vi "POST (Multipart).vi"(6 "timeout":i32=10000, 7 "output file":path, 8 "error in":errorcluster, 9 "data":T1[](array[typedef]), 10 "url":string, 11 "session in":refnum<class "Session.lvclass">) -> (0 "error out":errorcluster, 1 "body":string, 2 "headers":string, 3 "session out":refnum<class "Session.lvclass">, 4 "status code":u32)   [LabVIEW 2024, in "lib_NI_Advanced HTTP Client.lvlib" / "Session.lvclass"]
uses:
  Session.lvclass
  Multipart Data--cluster.ctl
  Session.lvclass/Session.ctl
  lvwebclient_64.dll
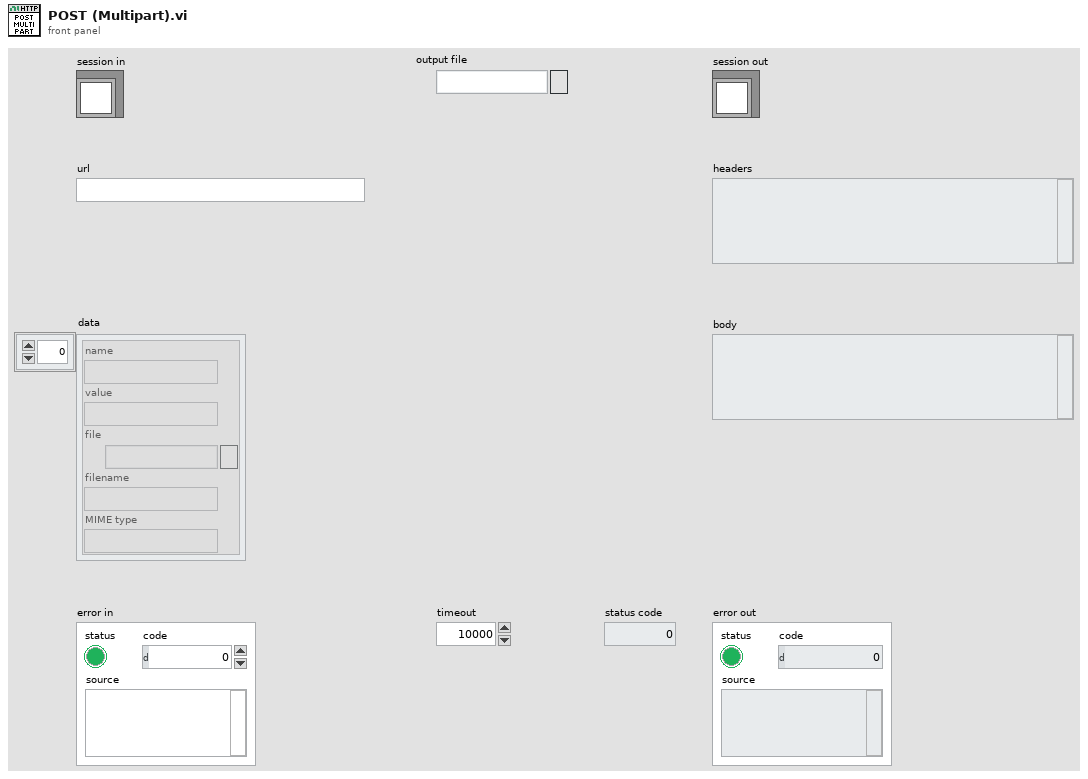
[diagram p1: front panel]
types:
  T1 = typedef "lib_NI_Advanced HTTP Client.lvlib/Session.lvclass/Multipart Data--cluster.ctl" = cluster{"name":string, "value":string, "file":path, "filename":string, "MIME type":string}
  T2 = cluster{"utf-8 text":string, "value":string, "file":path, "utf-8 text":string, "utf-8 text":string}
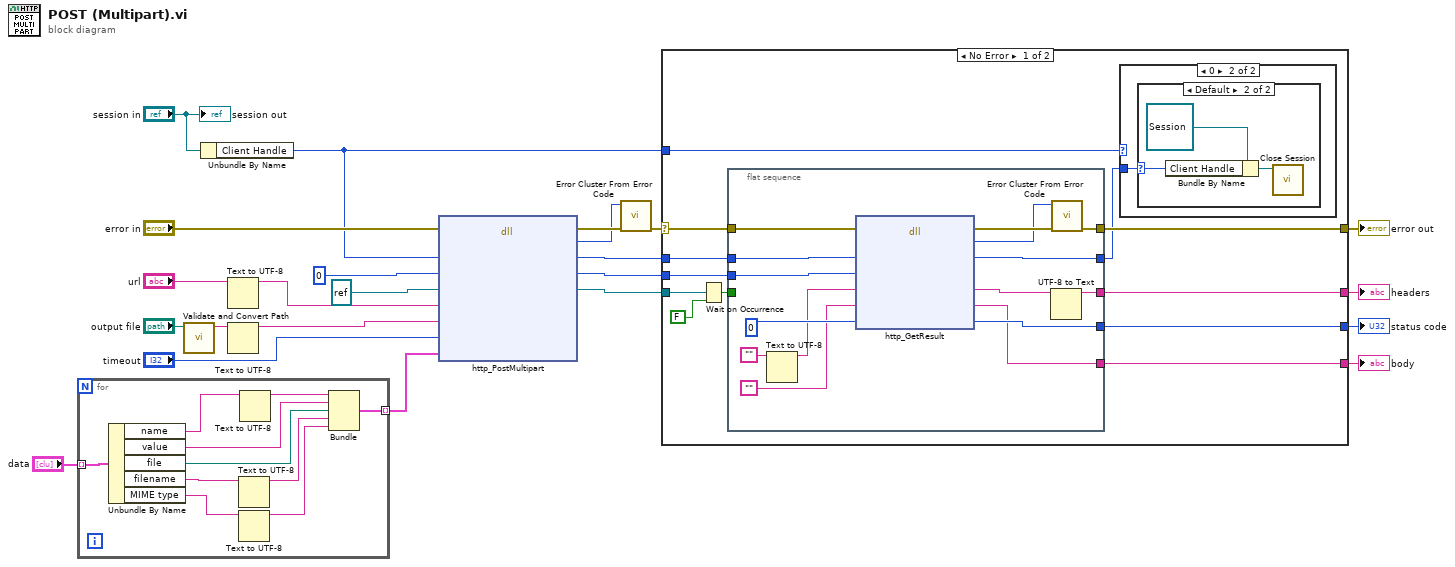
[diagram p0: block diagram]
diagram:
  n1 = for {
    tunnel: "data" -> [w33] mode=indexing
    tunnel: [w24] -> w1 mode=indexing
    n2 = Unbundle By Name(w33) -> ("name"=w32:string, "value"=w31:string, "file"=w29:path, "filename"=w28:string, "MIME type"=w26:string)
    n3 = Text to UTF-8(11:w28) -> (3:w27:string)  [unwired: 2 in, 1 out]
    n4 = Text to UTF-8(11:w26) -> (3:w25:string)  [unwired: 2 in, 1 out]
    n5 = Text to UTF-8(11:w32) -> (3:w30:string)  [unwired: 2 in, 1 out]
    n6 = Bundle("utf-8 text"=w30, "value"=w31, "file"=w29, "utf-8 text"=w27, "utf-8 text"=w25) -> (w24:T2)  [unwired: 1 in]
  }
  n7 = call "Validate and Convert Path.vi"("path"="output file") -> ("validated path as string"=w15:string)  [unwired: 10 in]
  n8 = Unbundle By Name("session in") -> ("Client Handle"=w11:u32)
  n9 = Text to UTF-8(11:"url") -> (3:w5:string)  [unwired: 2 in, 1 out]
  n10 = Text to UTF-8(11:w15) -> (3:w4:string)  [unwired: 2 in, 1 out]
  n11 = dll-call lib="C:/Program Files/National Instruments/LabVIEW 2024/vi.lib/NI/Advanced HTTP Client/lvwebclient_*.*" fn="http_PostMultipart"(error in="error in", "handle"=w11, "request"=u32 0, "completeOccurrence"=refnum<k4> refnum ("occurrence"), "url"=w5, "outPath"=w4, "timeout"="timeout", "postData"=w1) -> (error out=w13:errorcluster, "return"=w12:i32, "handle"=w9:u32, "request"=w8:u32, "completeOccurrence"=w6:refnum<k4>)  [unwired: 6 in, 1 out]
  n12 = call "Error Cluster From Error Code.vi"("error in (no error)"=w13, "error code (0)"=w12) -> ("error out"=w23:errorcluster)  [unwired: 7 in]
  n13 = case shown="No Error" w23 {
    selector: w23 -> [w43 w65]
    tunnel: w6 -> [w45 _]
    tunnel: w9 -> [w42 _]
    tunnel: w8 -> [w41 _]
    tunnel: [w40 _] -> w20
    tunnel: [w39 _] -> w19
    tunnel: [w38 _] -> w18
    tunnel: [w37 w65] -> w17
    tunnel: w11 -> [w36 _]
    frame No Error {
      n14 = Wait on Occurrence(1:FALSE, 2:w45) -> (0:w44:bool)  [unwired: 1 in]
      n15 = flat-sequence {
        tunnel: w44 -> [_]
        tunnel: w43 -> [w64]
        tunnel: w42 -> [w63]
        tunnel: w41 -> [w62]
        tunnel: [w60] -> w40
        tunnel: [w55] -> w39
        tunnel: [w56] -> w38
        tunnel: [w54] -> w37
        tunnel: [w53] -> w35
        frame #0 {
          n16 = Text to UTF-8(11:"") -> (3:w51:string)  [unwired: 2 in, 1 out]
          n17 = dll-call lib="C:/Program Files/National Instruments/LabVIEW 2024/vi.lib/NI/Advanced HTTP Client/lvwebclient_*.*" fn="http_GetResult"(error in=w64, "handle"=w63, "request"=w62, "returnHeader"=w51, "returnBody"="", "httpStatus"=u32 0) -> (error out=w59:errorcluster, "return"=w58:i32, "handle"=w53:u32, "returnHeader"=w57:string, "returnBody"=w56:string, "httpStatus"=w60:u32)  [unwired: 3 in, 1 out]
          n18 = UTF-8 to Text(11:w57) -> (3:w55:string)  [unwired: 2 in, 1 out]
          n19 = call "Error Cluster From Error Code.vi"("error in (no error)"=w59, "error code (0)"=w58) -> ("error out"=w54:errorcluster)  [unwired: 7 in]
        }
      }
      n20 = case shown="0" w36 {
        tunnel: w35 -> [_ w46]
        frame Default {
        }
        frame 0 {
          n21 = case shown="Default" w46 {
            selector: w46 -> [_ w49]
            frame 0 {
            }
            frame Default {
              n22 = Bundle By Name(cluster=refnum<class "Session.lvclass"> refnum ("NI_Advanced HTTP Client.lvlib:Session.lvclass"), "Client Handle"=w49) -> (w48:refnum<class "Session.lvclass">)
              n23 = call "Close Session.vi"("session"=w48) -> ()  [unwired: 10 in, 1 out]
            }
          }
        }
      }
    }
    frame Error {
    }
  }
  "error out" <- w17
  "headers" <- w19
  "body" <- w18
  "status code" <- w20
  "session out" <- "session in"
